vi "GetStatusLine.vi"(3 "Status":T1[](array[typedef])) -> (1 "Status":string)   [LabVIEW 2010]
uses:
  _ROSDefinition.vi
  MyState.ctl
panel:
  out "h(x)":i32[](array[numeric])
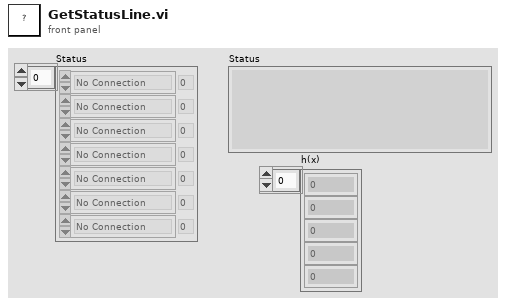
[diagram p1: front panel]
types:
  T1 = typedef "MyState.ctl" = enum16{"No Connection", "Registered", "Connected", "Close"}
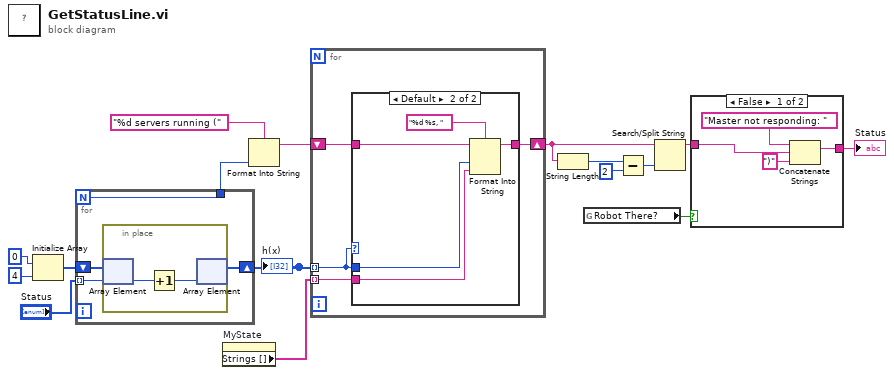
[diagram p0: block diagram]
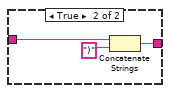
[diagram p2: hidden frame]
diagram:
  n1 = Initialize Array(u8 0 ("element"), 4 ("dimension size")) -> (w12:u8[])
  n2 = for {
    N -> [w17]
    shift-right: [w18] -> w8
    shift-left: w12 -> [w20]
    tunnel: "Status" -> [w19] mode=indexing
    tunnel: [w17] -> w2
    n3 = in-place {
      n4 = in-place-array #1(w20, w19) -> (w22:u8)
      n5 = Increment(x=w22) -> (x+1=w21:u8)
      n6 = in-place-array #1(w21) -> (w18:u8[])  [unwired: 1 out]
    }
  }
  "h(x)" <- w8
  n7 = property on="MyState" class="Enum (strict)"() -> ("Strings []"=w16:string[])  [unwired: 2 in, 2 out]
  n8 = Format Into String(format string="%d servers running (" ("regular expression"), w2) -> (resulting string=w13:string)  [unwired: 2 in, 1 out]
  n9 = for {
    shift-right: [w25] -> w6
    shift-left: w13 -> [w26]
    tunnel: w16 -> [w24] mode=indexing
    tunnel: w8 -> [w23] mode=indexing
    n10 = case shown="Default" w23 {
      tunnel: w26 -> [w27 w32]
      tunnel: [w27 w31] -> w25
      tunnel: w24 -> [_ w29]
      tunnel: w23 -> [_ w28]
      frame 0 {
      }
      frame Default {
        n11 = Format Into String(format string="%d %s, ", initial string=w32, w28, w29) -> (resulting string=w31:string)  [unwired: 1 in, 1 out]
      }
    }
  }
  n12 = String Length(string=w6) -> (length=w5:i32)
  n13 = global read "_ROSDefinition.vi" "Robot There?"() -> (w1:bool)
  n14 = Subtract(x=w5, y=2) -> (x-y=w3:i32)
  n15 = Search/Split String(string=w6, offset (0)=w3) -> (substring before match=w7:string)  [unwired: 1 in, 2 out]
  n16 = case shown="False" w1 {
    tunnel: [w34 w38] -> w15
    tunnel: w7 -> [w35 w37]
    frame False {
      n17 = Concatenate Strings("Master not responding: ", w35, ")" ("string")) -> (w34:string)
    }
    frame True {
      n18 = Concatenate Strings(w37, ")" ("string")) -> (w38:string)
    }
  }
  "Status" <- w15
